vi "FindIfActive.vi"(8 "error in (no error)":errorcluster, 10 "GUID":string, 11 "SMO.UI.MAUI in":refnum<class "SMO.UI.MAUI.lvclass">) -> (0 "error out":errorcluster, 1 "Panel":T1, 2 "Found?":bool, 3 "SMO.UI.MAUI out":refnum<class "SMO.UI.MAUI.lvclass">, 4 "Panel Index":i32)   [LabVIEW 2020, in "SMO.UI.MAUI.lvclass"]
uses:
  SMO.UI.MAUI.lvclass
  Typedefs/PanelData.ctl
  SMO.UI.MAUI.lvclass/SMO.UI.MAUI.ctl
  <vilib>/Levylab/SMO.UI.Embedded/SMO.UI.Embedded.lvclass
  C:/Program Files (x86)/National Instruments/LabVIEW 2020/vi.lib/JKI/JKI SMO/SMO/SMO.lvclass
  <vilib>/JKI/JKI SMO/SMO/SMO.lvclass
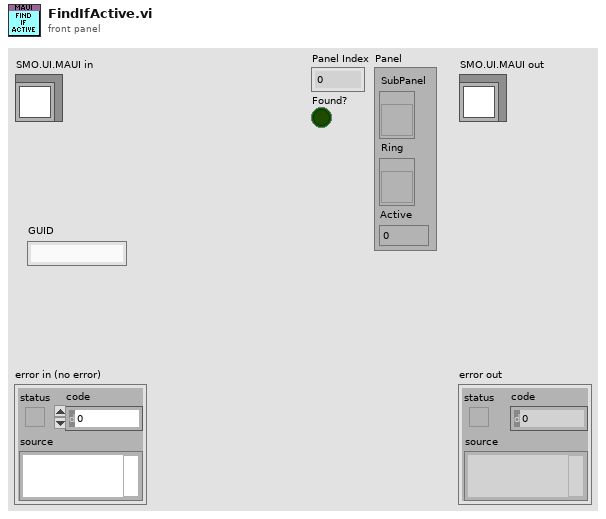
[diagram p1: front panel]
types:
  T1 = typedef "SMO.UI.MAUI.lvclass/PanelData.ctl" = cluster{"SubPanel":refnum<vi>, "Ring":refnum<vi>, "Active":i32}
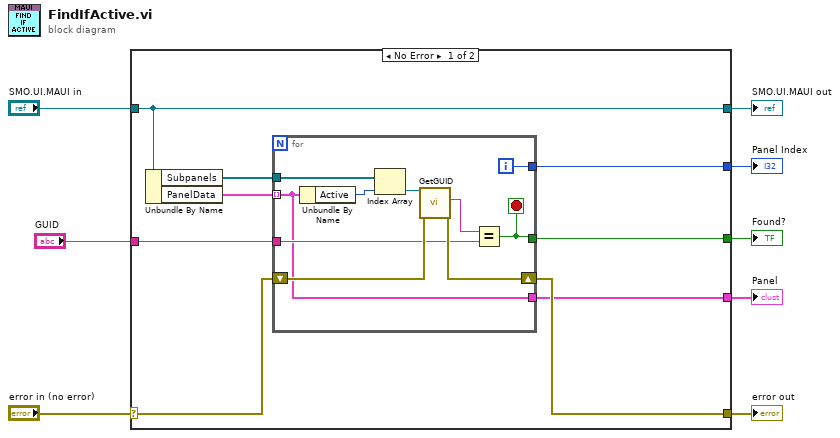
[diagram p0: block diagram]
diagram:
  n1 = case shown="No Error" "error in (no error)" {
    selector: "error in (no error)" -> [w13 w29]
    tunnel: [w12 w29] -> w7
    tunnel: [w17 w28] -> w5
    tunnel: "SMO.UI.MAUI in" -> [w17 w28]
    tunnel: "GUID" -> [w15 _]
    tunnel: [w11 _] -> w3
    tunnel: [w10 _] -> w2
    tunnel: [w9 _] -> w1
    frame No Error {
      n2 = Unbundle By Name(w17) -> ("Subpanels"=w16:refnum<class "SMO.UI.Embedded.lvclass">[], "PanelData"=w14:T1[])
      n3 = for {
        tunnel: w16 -> [w27]
        tunnel: w15 -> [w21]
        tunnel: w14 -> [w20] mode=indexing
        shift-right: [w23] -> w12
        shift-left: w13 -> [w24]
        tunnel: [w19] -> w11
        tunnel: [w20] -> w9
        tunnel: [w18] -> w10
        i -> [w18]
        stop <- w19 stop-if-true
        n4 = Unbundle By Name(w20) -> ("Active"=w26:i32)
        n5 = Index Array(array=w27, index=w26) -> (element=w25:refnum<class "SMO.UI.Embedded.lvclass">)
        n6 = call <vilib>:"GetGUID.vi"("error in (no error)"=w24, "SMO"=w25) -> ("error out"=w23:errorcluster, "GUID"=w22:string)  [unwired: 7 in, 1 out]
        n7 = Equal?(x=w22, y=w21) -> (x = y?=w19:bool)
      }
    }
    frame Error {
    }
  }
  "error out" <- w7
  "SMO.UI.MAUI out" <- w5
  "Panel Index" <- w2
  "Found?" <- w3
  "Panel" <- w1
